vi "ConfigureGroups.vi"(6 "all channels":T1[](array[typedef]), 8 "error in (no error)":errorcluster, 10 "acquisition channels (in acquisition order)":T1[](array[typedef]), 11 "device":T4) -> (0 "error out":errorcluster, 3 "groups":T11[](array[typedef]))   [LabVIEW 2017, in "McsaFpgaAcquisition.lvlib"]
uses:
  <vilib>/addons/InsightCM/Devices/Shared/Mcsa/McsaFpgaAcquisition/McsaFpgaAcquisition.lvlib
  <vilib>/addons/InsightCM/MessageBus/Base/controls/R2_Channel.ctl
  <vilib>/addons/InsightCM/MessageBus/Base/controls/KeyValuePair.ctl
  <vilib>/addons/InsightCM/MessageBus/Base/controls/Metric.ctl
  <vilib>/addons/InsightCM/Devices/Shared/Mcsa/McsaFpgaAcquisition/controls/Group.ctl
  <vilib>/addons/InsightCM/Devices/Shared/Mcsa/McsaFpgaAcquisition/controls/ChannelMcsa.ctl
  <vilib>/addons/InsightCM/Devices/Shared/Mcsa/McsaFpgaAcquisition/controls/RangeParams.ctl
  <vilib>/addons/InsightCM/MessageBus/Base/controls/R2_Device.ctl
  <vilib>/addons/InsightCM/MessageBus/Base/controls/DeviceState.ctl
  <vilib>/addons/InsightCM/MessageBus/Base/controls/R2_DataGroup.ctl
  <vilib>/addons/InsightCM/MessageBus/Base/controls/OperatingState.ctl
  <vilib>/addons/InsightCM/MessageBus/Base/controls/Trigger.ctl
  <vilib>/addons/InsightCM/MessageBus/Base/controls/Condition.ctl
  <vilib>/addons/InsightCM/MessageBus/Base/controls/BurstModeTrigger.ctl
  <vilib>/addons/InsightCM/MessageBus/Base/controls/R2_DeviceModel.ctl
  <vilib>/addons/InsightCM/MessageBus/Base/controls/Tag.ctl
  <vilib>/addons/InsightCM/Utilities/DeviceModelHelpers/DeviceModelHelpers.lvlib
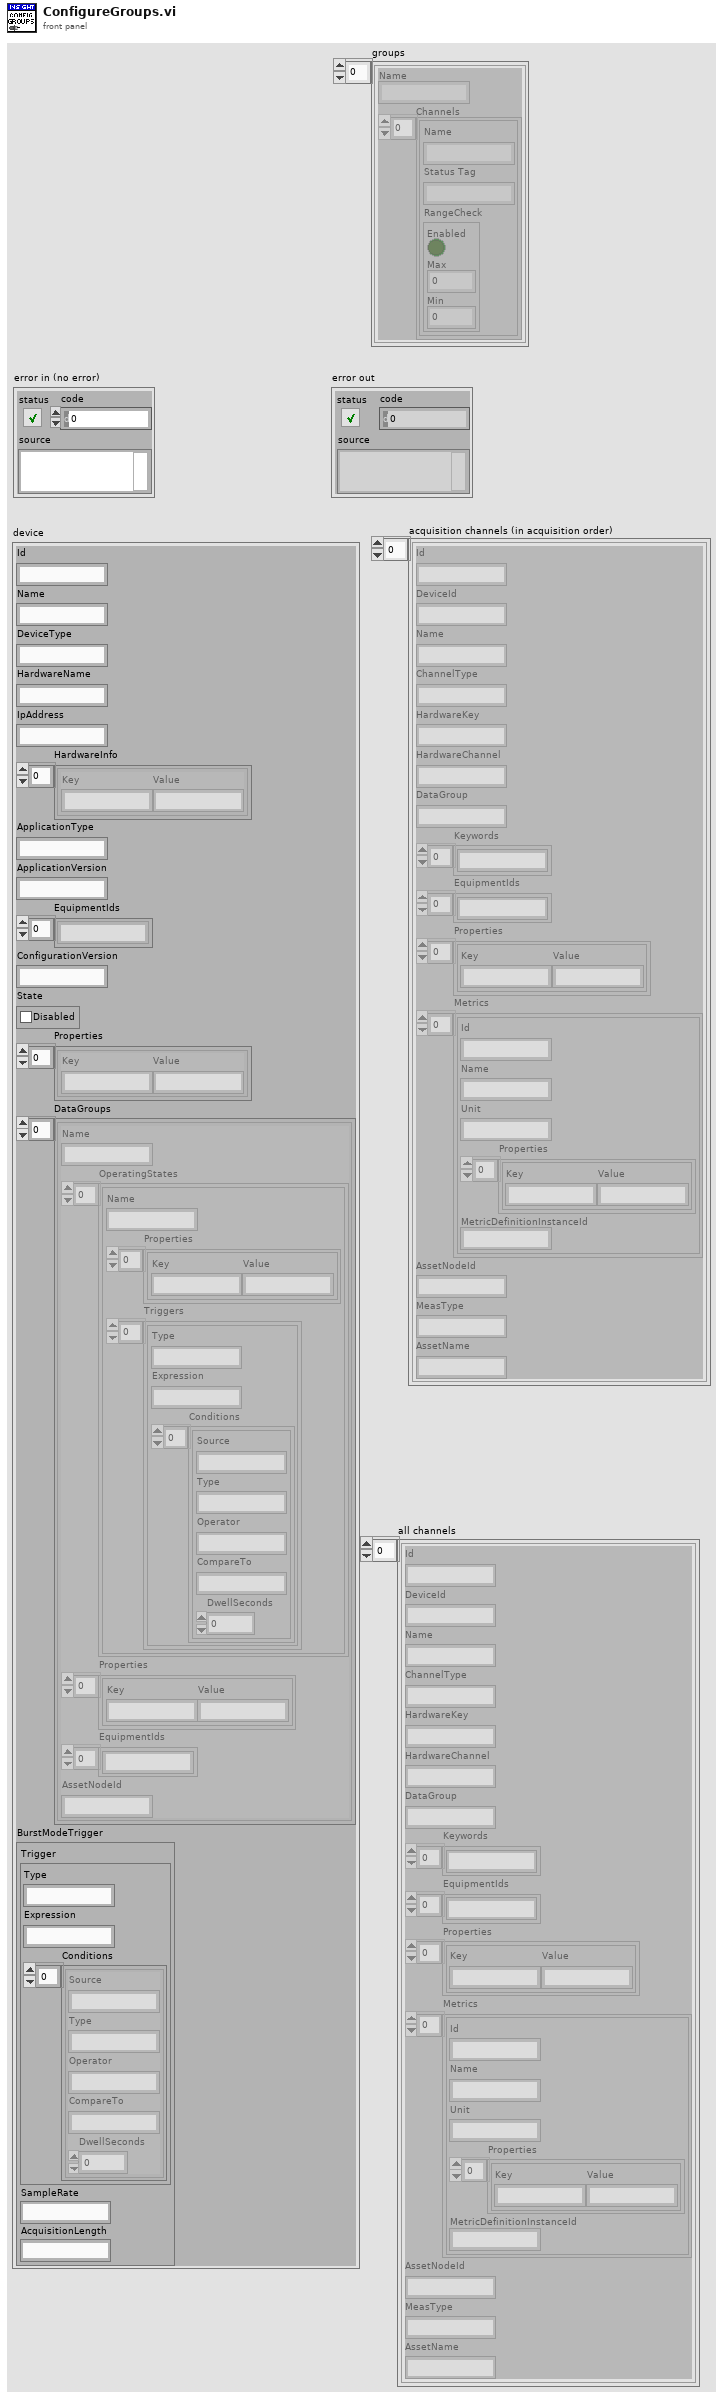
[diagram p1: front panel]
types:
  T1 = typedef "R2_Channel.ctl" = cluster{"Id":string, "DeviceId":string, "Name":string, "ChannelType":string, "HardwareKey":string, "HardwareChannel":string, "DataGroup":string, "Keywords":string[], "EquipmentIds":string[], "Properties":T2[], "Metrics":T3[], "AssetNodeId":string, "MeasType":string, "AssetName":string}
  T2 = typedef "KeyValuePair.ctl" = cluster{"Key":string, "Value":string}
  T3 = typedef "Metric.ctl" = cluster{"Id":string, "Name":string, "Unit":string, "Properties":T2[], "MetricDefinitionInstanceId":string}
  T4 = typedef "R2_Device.ctl" = cluster{"Id":string, "Name":string, "DeviceType":string, "HardwareName":string, "IpAddress":string, "HardwareInfo":T2[], "ApplicationType":string, "ApplicationVersion":string, "EquipmentIds":string[], "ConfigurationVersion":string, "State":T5, "Properties":T2[], "DataGroups":T6[], "BurstModeTrigger":T10}
  T5 = typedef "DeviceState.ctl" = cluster{"Disabled":bool}
  T6 = typedef "R2_DataGroup.ctl" = cluster{"Name":string, "OperatingStates":T7[], "Properties":T2[], "EquipmentIds":string[], "AssetNodeId":string}
  T7 = typedef "OperatingState.ctl" = cluster{"Name":string, "Properties":T2[], "Triggers":T8[]}
  T8 = typedef "Trigger.ctl" = cluster{"Type":string, "Expression":string, "Conditions":T9[]}
  T9 = typedef "Condition.ctl" = cluster{"Source":string, "Type":string, "Operator":string, "CompareTo":string, "DwellSeconds":dbl}
  T10 = typedef "BurstModeTrigger.ctl" = cluster{"Trigger":T8, "SampleRate":string, "AcquisitionLength":string}
  T11 = typedef "McsaFpgaAcquisition.lvlib/Group.ctl" = cluster{"Name":string, "Channels":T12[]}
  T12 = typedef "McsaFpgaAcquisition.lvlib/ChannelMcsa.ctl" = cluster{"Name":string, "Status Tag":string, "RangeCheck":T13}
  T13 = typedef "McsaFpgaAcquisition.lvlib/RangeParams.ctl" = cluster{"Enabled":bool, "Max":dbl, "Min":dbl}
  T14 = typedef "R2_DeviceModel.ctl" = cluster{"Device":T4, "Channels":T1[], "Tags":T15[]}
  T15 = typedef "Tag.ctl" = cluster{"Id":string, "Path":string, "Name":string, "Datatype":string, "Props":T2[], "Keywords":string[]}
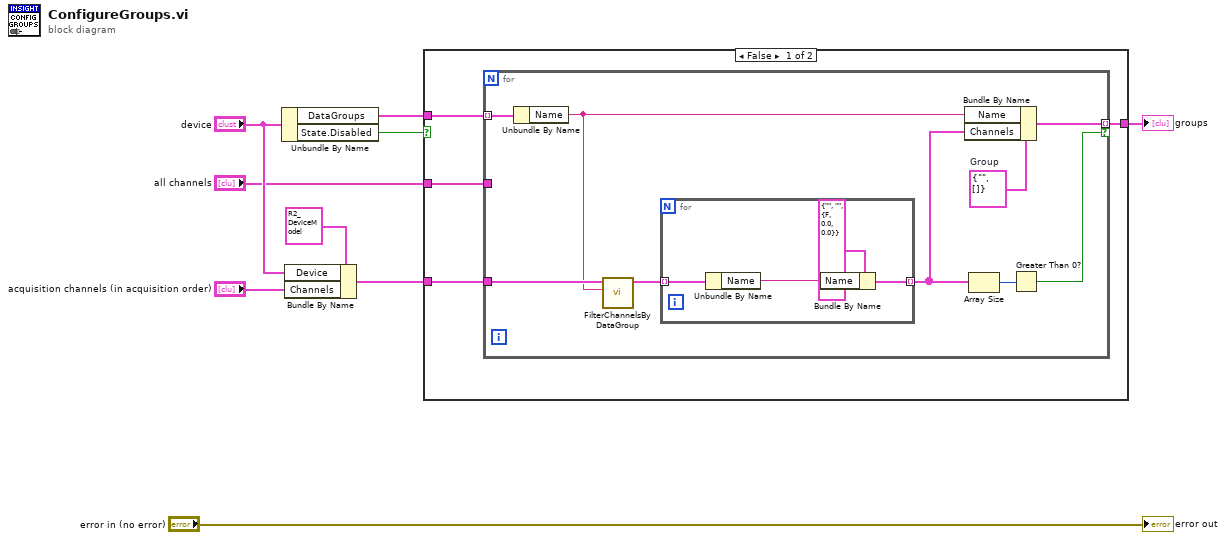
[diagram p0: block diagram]
diagram:
  n1 = Unbundle By Name("device") -> ("DataGroups"=w8:T6[], "State.Disabled"=w1:bool)
  n2 = Bundle By Name(cluster=T14 {"Device"={"Id"="", "Name"="", "DeviceType"="", "HardwareName"="", "IpAddress"="", "HardwareInfo"=[], "ApplicationType"="", "ApplicationVersion"="", "EquipmentIds"=[], "ConfigurationVersion"="", "State"={"Disabled"=FALSE}, "Properties"=[], "DataGroups"=[], "BurstModeTrigger"={"Trigger"={"Type"="", "Expression"="", "Conditions"=[]}, "SampleRate"="", "AcquisitionLength"=""}}, "Channels"=[], "Tags"=[]} ("device model"), "Device"="device", "Channels"="acquisition channels (in acquisition order)") -> (w4:T14)
  n3 = case shown="False" w1 {
    tunnel: [w13 _] -> w9
    tunnel: w8 -> [w12 _]
    tunnel: w4 -> [w11 _]
    tunnel: "all channels" -> [w10 _]
    frame False {
      n4 = for {
        tunnel: w12 -> [w22] mode=indexing
        tunnel: [w21] -> w13 mode=indexing if=w18
        tunnel: w11 -> [w17]
        tunnel: w10 -> [_]
        w14 = T11 {"Name"="", "Channels"=[]}  # Group
        n5 = Unbundle By Name(w22) -> ("Name"=w15:string)
        n6 = call <vilib>:"FilterChannelsByDataGroup.vi"("group"=w15, "device model"=w17) -> ("channels in data group"=w16:T1[])  [unwired: 8 in, 1 out]
        n7 = for {
          tunnel: [w26] -> w20 mode=indexing
          tunnel: w16 -> [w25] mode=indexing
          n8 = Unbundle By Name(w25) -> ("Name"=w23:string)
          n9 = Bundle By Name(cluster=T12 {"Name"="", "Status Tag"="", "RangeCheck"={"Enabled"=FALSE, "Max"=0.0, "Min"=0.0}} ("channel"), "Name"=w23) -> (w26:T12)
        }
        n10 = Bundle By Name(cluster=w14, "Name"=w15, "Channels"=w20) -> (w21:T11)
        n11 = Array Size(array=w20) -> (size(s)=w19:i32)
        n12 = Greater Than 0?(x=w19) -> (x > 0?=w18:bool)
      }
    }
    frame True {
    }
  }
  "groups" <- w9
  "error out" <- "error in (no error)"
